vi "CRC校验.vi"(8 "error in (no error)":errorcluster caption="错误输入（无错误）", 10 "puchMsg":string) -> (0 "error out":errorcluster caption="错误输出", 1 "CRC校验":string, 2 "数据段":string, 5 "数据段长度":string)   [LabVIEW 2016, in "中水三立SQL数据传输.lvlib" / "HJ212.lvclass"]
uses:
  HJ212.lvclass
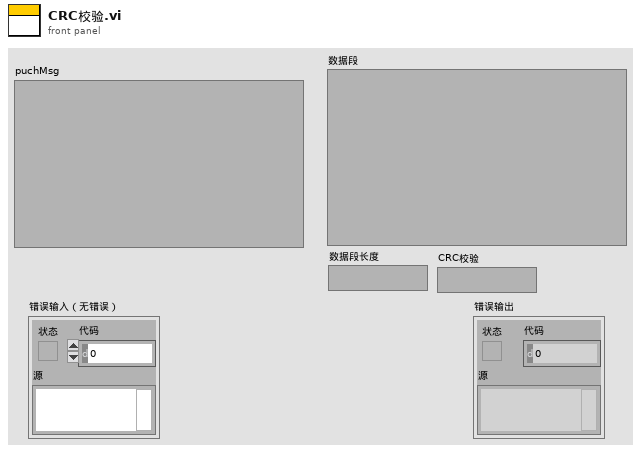
[diagram p1: front panel]
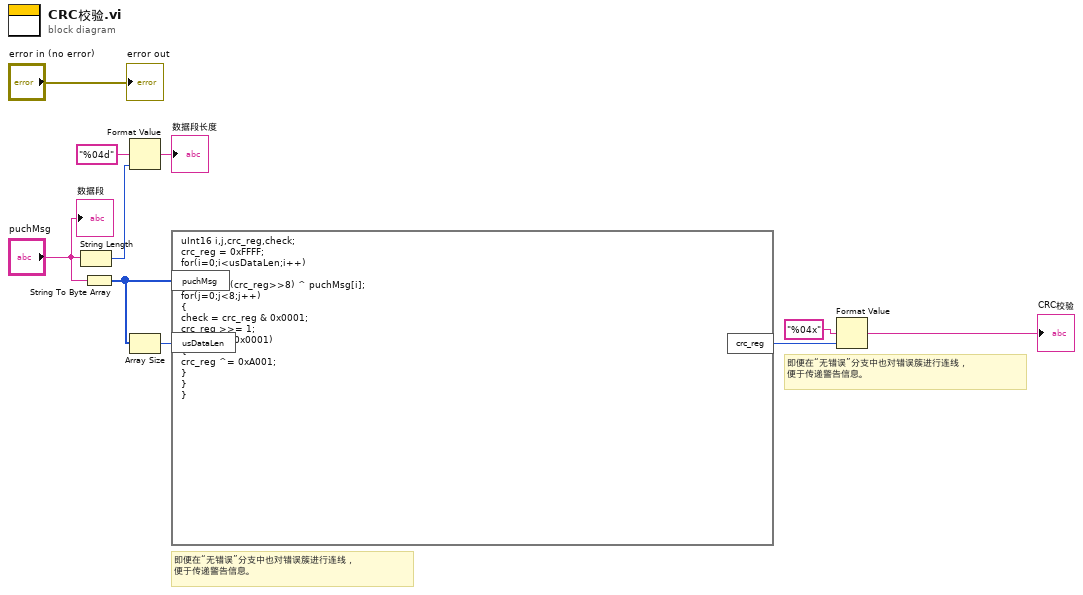
[diagram p0: block diagram]
diagram:
  # "即便在“无错误”分支中也对错误簇进行连线，\n便于传递警告信息。"
  # "即便在“无错误”分支中也对错误簇进行连线，\n便于传递警告信息。"
  n1 = String Length(string="puchMsg") -> (length=w4:i32)
  n2 = String To Byte Array(string="puchMsg") -> (unsigned byte array=w6:u8[])
  n3 = Format Value(format string="%04d" ("格式字符串"), value (0)=w4) -> (output string=→"数据段长度":string)  [unwired: 1 in]
  n4 = Array Size(array=w6) -> (size(s)=w5:i32)
  n5 = formula code="uInt16 i,j,crc_reg,check;\ncrc_reg = 0xFFFF;\nfor(i=0;i<usDataLen;i++)\n{\ncrc_reg = (crc_reg>>8) ^ puchMsg[i];\nfor(j=0;j<8;j++)\n{\ncheck = crc_reg & 0x0001;\ncrc_reg >>= 1;\nif(check==0x0001)\n{\ncrc_reg ^= 0xA001;\n}\n}\n}"("puchMsg"=w6, "usDataLen"=w5) -> ("crc_reg"=w1:u16)
  n6 = Format Value(format string="%04x" ("格式字符串"), value (0)=w1) -> (output string=→"CRC校验":string)  [unwired: 1 in]
  "error out" <- "error in (no error)"
  "数据段" <- "puchMsg"
